vi "Refresh Visible Size.vi"(8 "error in (no error)":errorcluster, 11 "2DArrayManager in":refnum<class "2DArrayManager.lvclass">) -> (0 "error out":errorcluster, 3 "2DArrayManager out":refnum<class "2DArrayManager.lvclass">)   [LabVIEW 2020, in "OOPanel.lvlib" / "2DArrayManager.lvclass"]
uses:
  2DArrayManager.lvclass
  2DArrayManager.lvclass/2DArrayManager.ctl
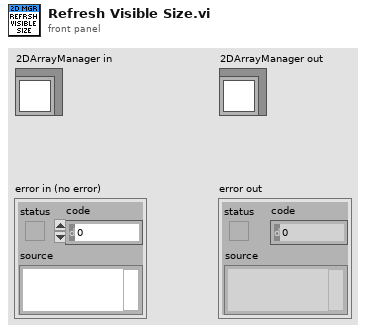
[diagram p1: front panel]
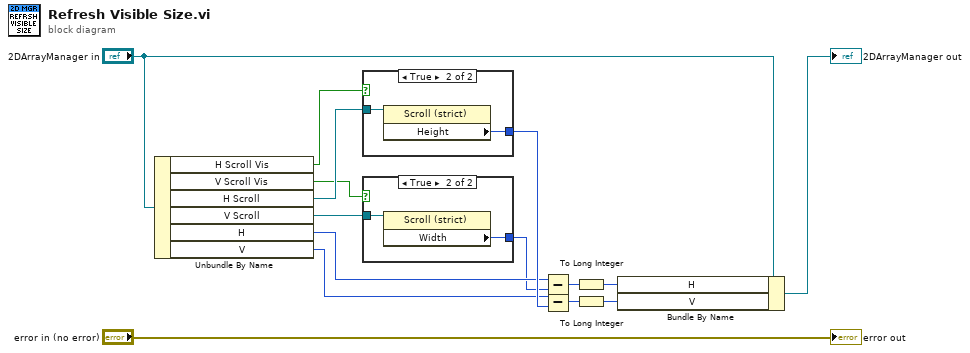
[diagram p0: block diagram]
diagram:
  n1 = Unbundle By Name("2DArrayManager in") -> ("H Scroll Vis"=w6:bool, "V Scroll Vis"=w3:bool, "H Scroll"=w12:refnum<vi>, "V Scroll"=w5:refnum<vi>, "H"=w8:i32, "V"=w7:i32)
  n2 = case shown="True" w6 {
    tunnel: w12 -> [_ w17]
    tunnel: [_ w16] -> w9
    frame False {
    }
    frame True {
      n3 = property class="Scroll (strict)"(reference=w17) -> ("Height"=w16:u32)  [unwired: 1 in, 2 out]
    }
  }
  n4 = case shown="True" w3 {
    tunnel: w5 -> [_ w19]
    tunnel: [_ w18] -> w4
    frame False {
    }
    frame True {
      n5 = property class="Scroll (strict)"(reference=w19) -> ("Width"=w18:u32)  [unwired: 1 in, 2 out]
    }
  }
  n6 = Subtract(x=w8, y=w4) -> (x-y=w11:u32)
  n7 = Subtract(x=w7, y=w9) -> (x-y=w10:u32)
  n8 = To Long Integer(number=w11) -> (32bit integer=w14:i32)
  n9 = To Long Integer(number=w10) -> (32bit integer=w13:i32)
  n10 = Bundle By Name(cluster="2DArrayManager in", "H"=w14, "V"=w13) -> (→"2DArrayManager out":refnum<class "2DArrayManager.lvclass">)
  "error out" <- "error in (no error)"
